vi "Bead tracking worker.vi"(6 "Bead tracking settings":T1, 7 "Worker index":u8, 8 "error in (no error)":errorcluster, 9 "Template":T2, 10 "Result queue":refnum<queue>, 11 "Data queue":refnum<queue>) -> ()   [LabVIEW 2011]
uses:
  TWOM-BeadTracking/Bead Tracking Mode.ctl
  Worker result.ctl
  <vilib>/vision/Image Controls.llb/IMAQ Image.ctl
  Bead tracking settings.ctl
  Worker data.ctl
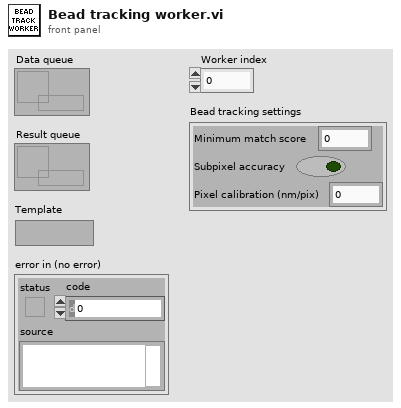
[diagram p1: front panel]
types:
  T1 = typedef "Bead tracking settings.ctl" = cluster{"Minimum match score":sgl, "Subpixel accuracy":bool, "Pixel calibration (nm/pix)":dbl}
  T2 = typedef "IMAQ Image.ctl" = refnum<image>
  T3 = typedef "Image Type" = u32
  T4 = typedef "Worker result.ctl" = cluster{"Index":u32, "Distance (um)":dbl, "Raw matches":cluster{"Position":cluster{"x":sgl, "y":sgl}, "Angle":sgl, "Scale":sgl, "Score":sgl, "Bounding Box":cluster{"x":sgl, "y":sgl}[]}[], "File":path}
  T5 = cluster{"left":i16, "top":i16, "right":i16, "bottom":i16}
  T6 = typedef "Worker data.ctl" = cluster{"Index":u32, "File":path}
  T7 = typedef "Bead Tracking Mode.ctl" = enum16{"Dual trap", "Q-trap =", "Q-trap ||", "Q-trap X", "Q-trap +", "Dual trap oO", "Single trap", "None"}
  T8 = cluster{"Position":cluster{"x":sgl, "y":sgl}, "Angle":sgl, "Scale":sgl, "Score":sgl, "Bounding Box":cluster{"x":sgl, "y":sgl}[]}[]
  T9 = typedef "Bead Tracking Matches.ctl" = cluster{"Bead 1 x":dbl, "Bead 1 y":dbl, "Bead 2 x":dbl, "Bead 2 y":dbl}[]
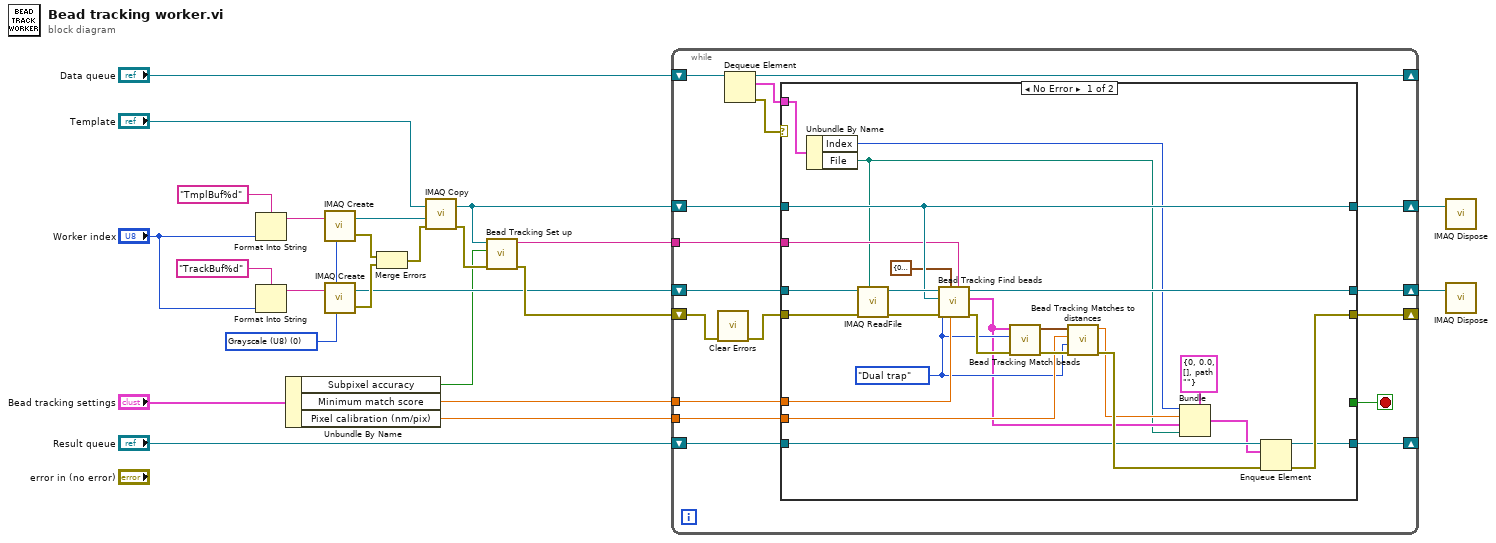
[diagram p0: block diagram]
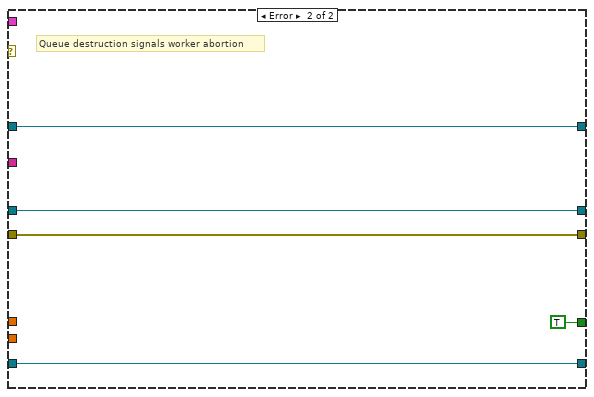
[diagram p2: hidden frame]
diagram:
  w14 = T3 0 items=["Grayscale (U8)", "Grayscale (I16)", "Grayscale (SGL)", "Complex (CSG)", "RGB (U32)", "HSL (U32)", "RGB (U64)", "Grayscale (U16)"] ("Image Type")
  n1 = Format Into String(format string="TmplBuf%d", "Worker index") -> (resulting string=w16:string)  [unwired: 2 in, 1 out]
  n2 = Format Into String(format string="TrackBuf%d", "Worker index") -> (resulting string=w15:string)  [unwired: 2 in, 1 out]
  n3 = Unbundle By Name("Bead tracking settings") -> ("Subpixel accuracy"=w5:bool, "Minimum match score"=w3:sgl, "Pixel calibration (nm/pix)"=w2:dbl)
  n4 = call "IMAQ Create"("Image Name"=w16, "Image Type"=w14) -> ("New Image"=w12:T2, "error out"=w24:errorcluster)  [unwired: 3 in]
  n5 = call "IMAQ Create"("Image Name"=w15, "Image Type"=w14) -> ("New Image"=w10:T2, "error out"=w23:errorcluster)  [unwired: 3 in]
  n6 = Merge Errors(w24, w23) -> (w22:errorcluster)
  n7 = call "IMAQ Copy"("error in (no error)"=w22, "Image Dst"=w12, "Image Src"="Template") -> ("error out"=w21:errorcluster, "Image Dst Out"=w7:T2)  [unwired: 3 in]
  n8 = call "Bead Tracking Set up.vi"("error in (no error)"=w21, "SubPixel Accuracy"=w5, "Template"=w7) -> ("error out"=w20:errorcluster, "Match Pattern Setup Data"=w4:string)  [unwired: 7 in]
  n9 = while {
    shift-right: [w36] -> w9
    shift-left: w7 -> [w35]
    shift-right: [w32] -> _
    shift-left: "Data queue" -> [w38]
    shift-right: [w34] -> w8
    shift-left: w10 -> [w33]
    tunnel: w4 -> [w30]
    shift-right: [w39] -> _
    shift-left: w20 -> [w40]
    tunnel: w3 -> [w29]
    tunnel: w2 -> [w28]
    shift-right: [w26] -> _
    shift-left: "Result queue" -> [w27]
    stop <- w37 stop-if-true
    n10 = call <vilib>:"Clear Errors.vi"("error in (no error)"=w40) -> ("error out"=w25:errorcluster)  [unwired: 6 in]
    n11 = Dequeue Element(queue=w38) -> (queue out=w32:refnum<queue>, element=w31:T6, error out=w41:errorcluster)  [unwired: 2 in, 1 out]
    n12 = case shown="No Error" w41 {
      tunnel: [_ TRUE] -> w37
      tunnel: [w56 w69] -> w36
      tunnel: w35 -> [w56 w69]
      tunnel: [w57 w68] -> w34
      tunnel: w33 -> [w59 w68]
      tunnel: w31 -> [w60 _]
      tunnel: w30 -> [w55 _]
      tunnel: w25 -> [w65 w71]
      tunnel: [w61 w71] -> w39
      tunnel: w29 -> [w53 _]
      tunnel: w28 -> [w52 _]
      tunnel: w27 -> [w50 w67]
      tunnel: [w49 w67] -> w26
      frame No Error {
        w51 = Bead_Tracking_Mode."Dual trap" ("Bead Tracking Mode")
        n13 = Unbundle By Name(w60) -> ("Index"=w47:u32, "File"=w42:path)
        n14 = call "IMAQ ReadFile"("File Path"=w42, "error in (no error)"=w65, "Image"=w59) -> ("error out"=w66:errorcluster, "Image Out"=w58:T2)  [unwired: 4 in, 3 out]
        n15 = call "Bead Tracking Find beads.vi"("Match Pattern Setup Data"=w55, "Minimum Match Score"=w53, "Search Rectangle"=T5 {"left"=0, "top"=0, "right"=0, "bottom"=0}, "error in (no error)"=w66, "Bead Tracking Mode"=w51, "Template"=w56, "Image"=w58) -> ("error out"=w64:errorcluster, "Raw matches"=w43:T8, "Image out"=w57:T2)  [unwired: 1 in, 1 out]
        n16 = call "Bead Tracking Match beads.vi"("error in (no error)"=w64, "Bead Tracking Mode"=w51, "Raw Matches"=w43) -> ("error out"=w63:errorcluster, "Bead Tracking Matches"=w45:T9)  [unwired: 7 in]
        n17 = call "Bead Tracking Matches to distances.vi"("error in (no error)"=w63, "Bead Tracking Mode"=w51, "Distance calibration (nm/pix)"=w52, "Matches"=w45) -> ("error out"=w62:errorcluster, "Distance 1 (um)"=w46:dbl)  [unwired: 4 in, 2 out]
        n18 = Bundle(cluster=T4 {"Index"=0, "Distance (um)"=0.0, "Raw matches"=[], "File"=path ""} ("Worker result"), "Index"=w47, "Distance (um)"=w46, "Raw matches"=w43, "File"=w42) -> (w44:T4)
        n19 = Enqueue Element(queue=w50, element=w44, error in (no error)=w62) -> (queue out=w49:refnum<queue>, error out=w61:errorcluster)  [unwired: 1 in, 1 out]
      }
      frame Error {
        # "Queue destruction signals worker abortion"
      }
    }
  }
  n20 = call "IMAQ Dispose"("Image"=w9) -> ()  [unwired: 5 in, 1 out]
  n21 = call "IMAQ Dispose"("Image"=w8) -> ()  [unwired: 5 in, 1 out]
